vi "Test Resize Greyscale.vi"(8 "error in (no error)":errorcluster, 11 "Test Case In":refnum<class "01_Image.lvclass">) -> (0 "error out":errorcluster, 3 "Test Case Out":refnum<class "01_Image.lvclass">)   [LabVIEW 2020, in "test.lvlib" / "01_Image.lvclass"]
uses:
  01_Image.lvclass
  C:/Program Files (x86)/National Instruments/LabVIEW 2026/vi.lib/Astemes/LUnit/Test Case.lvclass
  common/Image Size (Integer).ctl
  image/Interpolation Mode.ctl
  <vilib>/Astemes/LUnit/Test Case.lvclass/Test Case.ctl
  image/New Image (Greyscale Preallocated).vi
  image/Resize (Greyscale).vi
  4993e8ee-a06a-463a-9684-69129f64d5ce.vi
  image/Copy Array to Image.vi
  image/Copy Array to Image (Greyscale).vi
  image/New Image (Greyscale Preallocated).vi/6598b9e0-8a08-46f5-91fd-ca1b87217137.vi
  image/Resize (Greyscale).vi/eaa3f26c-b51e-4a69-9610-cf2aa5919b39.vi
  <vilib>/Astemes/LUnit/Core/LUnit Test Case/Private/Append Pass Result.vi
  <vilib>/Astemes/LUnit/Core/LUnit Test Case/Private/Append Fail Result.vi
  4993e8ee-a06a-463a-9684-69129f64d5ce.vi/9c5d11cd-9439-4240-a1ee-d9baace9c924.vi
  <vilib>/Astemes/LUnit/Core/LUnit Test Case/Private/Run In UI.vi
  <vilib>/Utility/error.llb/Clear Errors.vi
  <vilib>/Utility/error.llb/Error Cluster From Error Code.vi
  <vilib>/picture/pixmap.llb/Flatten Pixmap.vi
  image/image.lvlib
  common/common.lvlib
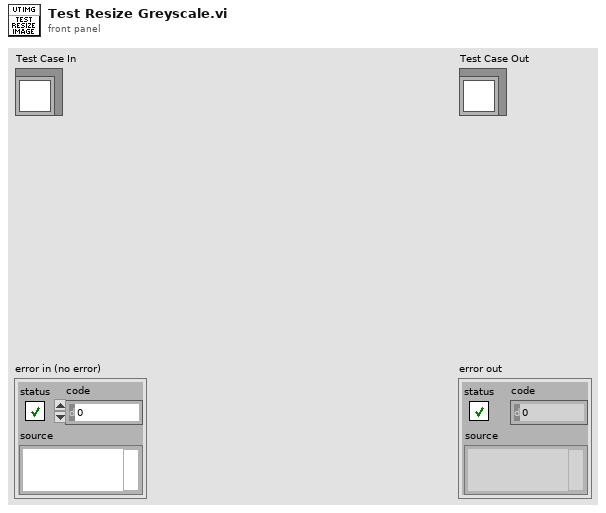
[diagram p1: front panel]
types:
  T1 = typedef "image.lvlib/Interpolation Mode.ctl" = enum8{"NEAREST", "LINEAR", "CUBIC", "AREA", "LANCZOS", "LINEAR_EXACT", "NEAREST_EXACT", "MAX"}
  T2 = typedef "common.lvlib/Image Size (Integer).ctl" = cluster{"Width":u16, "Height":u16}
  T3 = typedef "image.lvlib/Greyscale Image.ctl" = refnum<data-value>
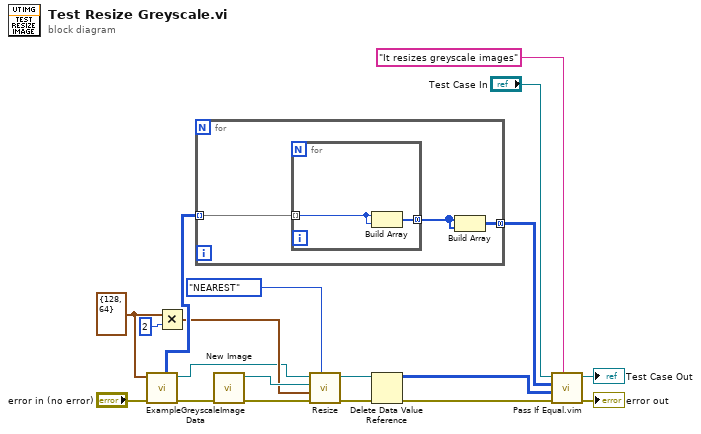
[diagram p0: block diagram]
diagram:
  w5 = T2 {"Width"=128, "Height"=64} ("Preallocated Image Size (Default - 0,0)")
  n1 = call "ExampleGreyscaleImageData.vi"("error in (no error)"="error in (no error)", "Image Size"=w5) -> ("error out"=w1:errorcluster, "Greyscale Destination Image"=w3:T3, "Greyscale Data"=w10:u8[][])  [unwired: 6 in, 1 out]
  n2 = Multiply(x=w5, y=u16 2) -> (x*y=w4:T2)
  n3 = for {
    tunnel: w10 -> [w22] mode=indexing
    tunnel: [w20] -> w9 mode=concatenating
    n4 = for {
      tunnel: w22 -> [w24] mode=indexing
      tunnel: [w23] -> w21 mode=concatenating
      n5 = Build Array(w24, w24) -> (w23:u8[])
    }
    n6 = Build Array(w21, w21) -> (w20:u8[][])
  }
  n7 = call-poly "New Image.vi"("error in (no error)"=w1) -> ("error out"=w7:errorcluster, "Greyscale Image"=w6:T3)  [unwired: 9 in]
  n8 = call-poly "Resize.vi"("Interpolation Mode (Default: CUBIC)"=Interpolation_Mode."NEAREST" ("OpenCV Interpolation Flag"), "error in (no error)"=w7, "New Image Size"=w4, "Greyscale Destination Image in"=w6, "Greyscale Source Image in"=w3) -> ("error out"=w12:errorcluster, "Greyscale Destination Image"=w13:T3)  [unwired: 5 in]
  n9 = Delete Data Value Reference(data value reference=w13, error in=w12) -> (data value=w14:u8[][], error out=w16:errorcluster)
  n10 = call "Pass If Equal.vim"("Description"="It resizes greyscale images", "error in (no error)"=w16, "Actual"=w14, "Expected"=w9, "LUnit Test Case In"="Test Case In") -> ("error out"=→"error out":errorcluster, "LUnit Test Case Out"=→"Test Case Out":refnum<class "01_Image.lvclass">)  [unwired: 5 in]
